vi "Load Questions from Disk.vi"(8 "error in (no error)":errorcluster, 10 "Path":path, 11 "Controller in":refnum<class "Controller.lvclass">) -> (0 "error out":errorcluster, 3 "Controller out":refnum<class "Controller.lvclass">)   [LabVIEW 2021, in "Controller.lvlib" / "Controller.lvclass"]
uses:
  Controller.lvclass
  Controller.lvclass/Controller.ctl
  <userlib>/_OpenG.lib/file/file.llb/Strip Path Extension - Path__ogtk.vi
  <userlib>/_OpenG.lib/file/file.llb/File Exists - Scalar__ogtk.vi
  <userlib>/_OpenG.lib/file/file.llb/Convert File Extension (Path)__ogtk.vi
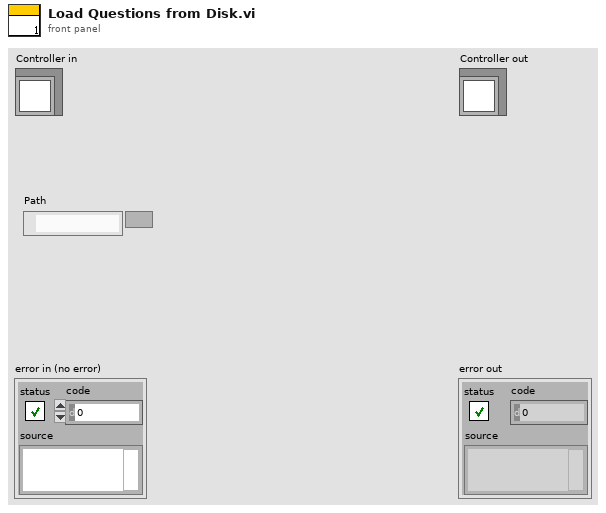
[diagram p1: front panel]
types:
  T1 = map{cluster{"String":string, "String":string}, path}
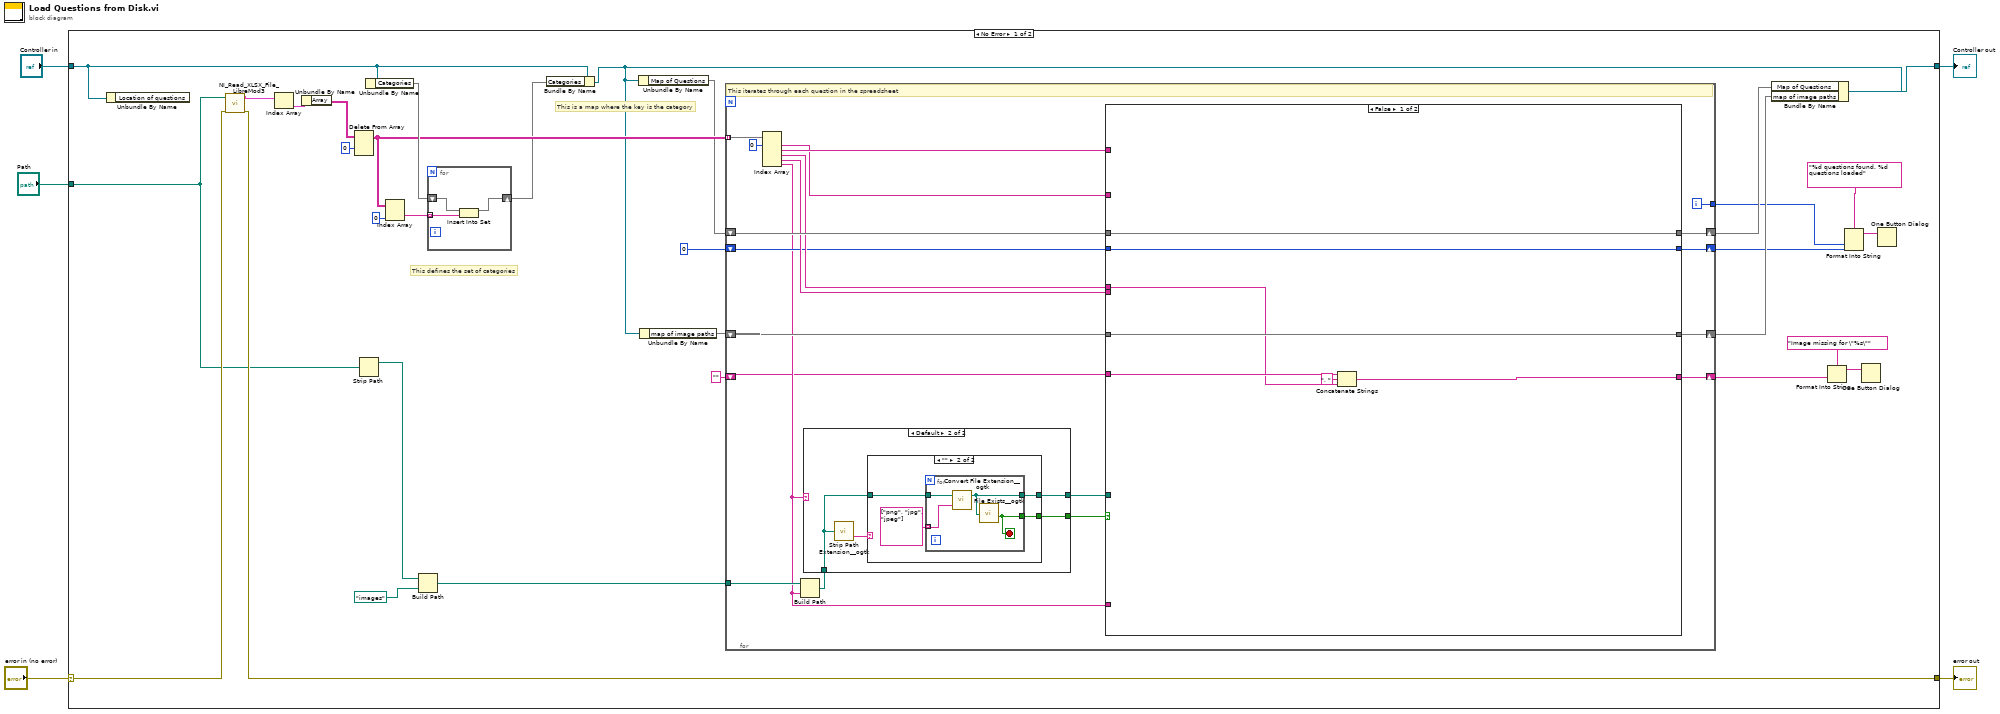
[diagram p0: block diagram]
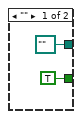
[diagram p2: hidden frame]
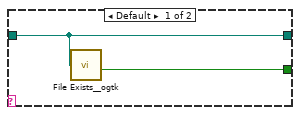
[diagram p3: hidden frame]
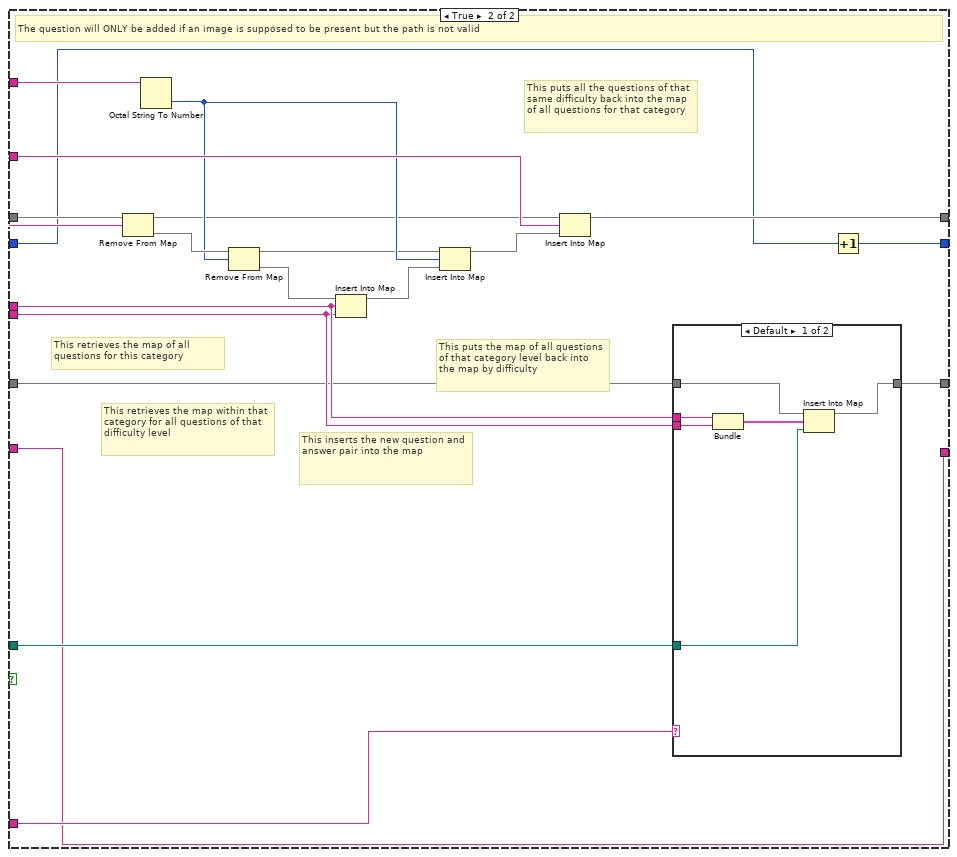
[diagram p4: hidden frame]
diagram:
  n1 = case shown="No Error" "error in (no error)" {
    selector: "error in (no error)" -> [w21 w111]
    tunnel: [w20 w111] -> w4
    tunnel: [w26 w110] -> w2
    tunnel: "Controller in" -> [w30 w110]
    tunnel: "Path" -> [w15 _]
    frame No Error {
      # "This is a map where the key is the category"
      # "This defines the set of categories"
      n2 = Unbundle By Name(w30) -> ()  [unwired: 1 out]
      n3 = call "NI_Read_XLSX_File_LibreMod3.vi"("error in"=w21, "XLSX File"=w15) -> ("error out"=w20:errorcluster, "Sheet Data"=w19:cluster{"Array":string[][]}[])  [unwired: 7 in, 1 out]
      n4 = Index Array(array=w19) -> (element=w36:cluster{"Array":string[][]})  [unwired: 1 in]
      n5 = Unbundle By Name(w36) -> ("Array"=w35:string[][])
      n6 = Delete From Array(array=w35, index (row)=0) -> (array with subset deleted=w29:string[][])  [unwired: 2 in, 1 out]
      n7 = Strip Path(path=w15) -> (stripped path=w18:path)  [unwired: 1 out]
      n8 = Unbundle By Name(w30) -> ("Categories"=w31:set{string})
      n9 = Index Array(array=w29, index (col)=0 ("disabled index (col)")) -> (element=w32:string[])  [unwired: 1 in]
      n10 = Build Path(base path=w18, name or relative path=path "images") -> (appended path=w16:path)
      n11 = for {
        tunnel: w32 -> [w109] mode=indexing
        shift-right: [w108] -> w28
        shift-left: w31 -> [w107]
        n12 = Insert Into Set(10:w109, 11:w107) -> (3:w108:set{string})  [unwired: 1 out]
      }
      n13 = Bundle By Name(cluster=w30, "Categories"=w28) -> (w23:refnum<class "Controller.lvclass">)
      n14 = Unbundle By Name(w23) -> ("Map of Questions"=w27:map{string, map{u32, map{string, string}}})
      n15 = Unbundle By Name(w23) -> ("map of image paths"=w22:T1)
      n16 = for {
        tunnel: w29 -> [w56] mode=indexing
        shift-right: [w53] -> w25
        shift-left: w27 -> [w51]
        shift-right: [w48] -> w24
        shift-left: w22 -> [w47]
        tunnel: w16 -> [w45]
        tunnel: [w46] -> w12
        shift-right: [w44] -> w10
        shift-left: 0 ("input 2") -> [w43]
        shift-right: [w38] -> w6
        shift-left: "" -> [w37]
        i -> [w46]
        # "This iterates through each question in the spreadsheet"
        n17 = Index Array(array=w56, index #1=0 ("index")) -> (element #1=w52:string, element #2=w54:string, element #3=w50:string, element #4=w49:string, element #5=w39:string)  [unwired: 4 in]
        n18 = Build Path(base path=w45, name or relative path=w39) -> (appended path=w42:path)
        n19 = case shown="Default" w39 {
          tunnel: w42 -> [_ w61]
          tunnel: [TRUE ("exists") w60] -> w41
          tunnel: [path "" ("new filename") w59] -> w40
          frame "" {
          }
          frame Default {
            n20 = call-poly <userlib>:"Strip Path Extension__ogtk.vi"("path"=w61) -> ("extension"=w62:string)  [unwired: 1 out]
            n21 = case shown="\"\"" w62 {
              tunnel: w61 -> [w64 w67]
              tunnel: [w64 w66] -> w59
              tunnel: [w63 w65] -> w60
              frame Default {
                n22 = call-poly <userlib>:"File Exists__ogtk.vi"("file path"=w64) -> ("exists"=w63:bool)  [unwired: 6 in, 1 out]
              }
              frame "" {
                n23 = for {
                  tunnel: string[] ["png", "jpg", "jpeg"] -> [w72] mode=indexing
                  tunnel: w67 -> [w71]
                  tunnel: [w70] -> w66
                  tunnel: [w69] -> w65
                  stop <- w69 stop-if-true
                  n24 = call-poly <userlib>:"Convert File Extension__ogtk.vi"("new ending (none)"=w72, "file name"=w71) -> ("new filename"=w70:path)  [unwired: 1 out]
                  n25 = call-poly <userlib>:"File Exists__ogtk.vi"("file path"=w70) -> ("exists"=w69:bool)  [unwired: 6 in, 1 out]
                }
              }
            }
          }
        }
        n26 = case shown="False" w41 {
          tunnel: w54 -> [_ w99]
          tunnel: [w79 w96] -> w53
          tunnel: w52 -> [_ w95]
          tunnel: w51 -> [w79 w94]
          tunnel: w50 -> [w74 w88]
          tunnel: w49 -> [_ w87]
          tunnel: [w78 w86] -> w48
          tunnel: w47 -> [w78 w85]
          tunnel: w39 -> [_ w84]
          tunnel: [w77 w82] -> w44
          tunnel: w43 -> [w77 w83]
          tunnel: w40 -> [_ w81]
          tunnel: [w76 w80] -> w38
          tunnel: w37 -> [w75 w80]
          frame False {
            n27 = Concatenate Strings(w75, ", " ("string"), w74) -> (w76:string)
          }
          frame True {
            # "This puts all the questions of that same difficulty back into the map of all questions for that category"
            # "This puts the map of all questions of that category level back into the map by difficulty"
            # "This inserts the new question and answer pair into the map"
            # "This retrieves the map within that category for all questions of that difficulty level"
            # "This retrieves the map of all questions for this category"
            # "The question will ONLY be added if an image is supposed to be present but the path is not valid"
            n28 = Remove From Map(10:w95, 11:w94) -> (1:w93:map{u32, map{string, string}}, 3:w89:map{string, map{u32, map{string, string}}})  [unwired: 1 out]
            n29 = Octal String To Number(4:w99) -> (0:w92:u32)  [unwired: 2 in, 1 out]
            n30 = Remove From Map(10:w92, 11:w93) -> (1:w91:map{string, string}, 3:w90:map{u32, map{string, string}})  [unwired: 1 out]
            n31 = Insert Into Map(map in=w91, key=w88, value=w87) -> (map out=w98:map{string, string})  [unwired: 2 out]
            n32 = Insert Into Map(map in=w90, key=w92, value=w98) -> (map out=w97:map{u32, map{string, string}})  [unwired: 2 out]
            n33 = Insert Into Map(map in=w89, key=w95, value=w97) -> (map out=w96:map{string, map{u32, map{string, string}}})  [unwired: 2 out]
            n34 = case shown="Default" w84 {
              tunnel: w88 -> [w105 _]
              tunnel: w87 -> [w104 _]
              tunnel: [w102 w106] -> w86
              tunnel: w85 -> [w101 w106]
              tunnel: w81 -> [w100 _]
              frame Default {
                n35 = Bundle("String"=w105, "String"=w104) -> (w103:cluster{"String":string, "String":string})  [unwired: 1 in]
                n36 = Insert Into Map(map in=w101, key=w103, value=w100) -> (map out=w102:T1)  [unwired: 2 out]
              }
              frame "" {
              }
            }
            n37 = Increment(x=w83) -> (x+1=w82:i32)
          }
        }
      }
      n38 = Bundle By Name(cluster=w23, "Map of Questions"=w25, "map of image paths"=w24) -> (w26:refnum<class "Controller.lvclass">)
      n39 = Format Into String(format string="Image missing for \"%s\"", w6) -> (resulting string=w8:string)  [unwired: 2 in, 1 out]
      n40 = Format Into String(format string="%d questions found. %d questions loaded", w12, w10) -> (resulting string=w14:string)  [unwired: 2 in, 1 out]
      n41 = One Button Dialog(message=w8) -> ()  [unwired: 1 in, 1 out]
      n42 = One Button Dialog(message=w14) -> ()  [unwired: 1 in, 1 out]
    }
    frame Error {
    }
  }
  "error out" <- w4
  "Controller out" <- w2
